vi "get_zero_crossings.vi"(9 "signal":dbl[](array[numeric]), 10 "index":dbl[](array[numeric])) -> (0 "size of p->n array":i32, 1 "size of n->p array":i32, 2 "p->n indexes":i32[](array[numeric]), 3 "n->p indexes":i32[](array[numeric]))   [LabVIEW 2019]
uses:
  <vilib>/ptbypt/NI_PtbyPt.lvlib
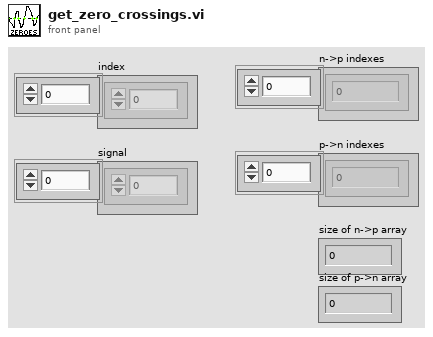
[diagram p1: front panel]
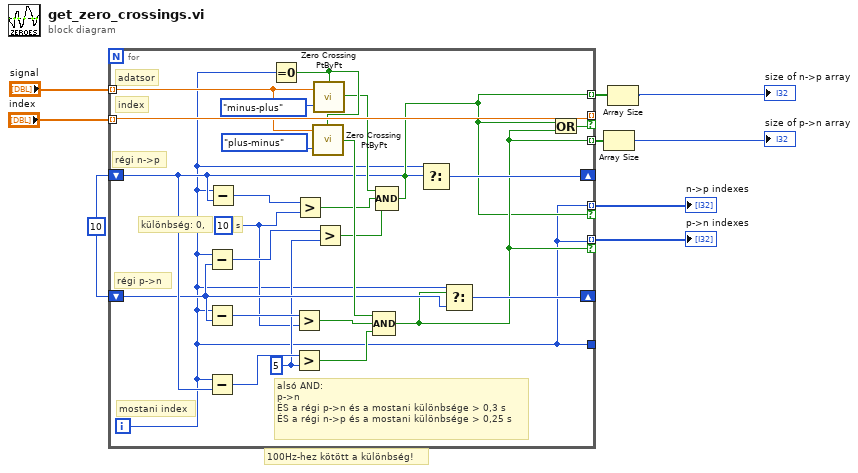
[diagram p0: block diagram]
diagram:
  w5 = 10
  # "100Hz-hez kötött a különbség!"
  n1 = for {
    tunnel: "signal" -> [w33] mode=indexing
    tunnel: "index" -> [w34] mode=indexing
    tunnel: [w34] -> _ mode=indexing if=w25
    tunnel: [w12] -> w2 mode=indexing
    tunnel: [w11] -> w6 mode=indexing
    shift-right: [w30] -> _
    shift-left: w5 -> [w21]
    shift-right: [w29] -> _
    shift-left: w5 -> [w17]
    tunnel: [w10] -> w7 mode=indexing if=w11
    tunnel: [w10] -> w8 mode=indexing if=w12
    tunnel: [w10] -> _
    i -> [w10]
    w14 = 5 ("y")
    w13 = 10
    # "adatsor"
    # "régi p->n"
    # "régi n->p"
    # "index"
    # "alsó AND:\np->n\nÉS a régi p->n és a mostani különbsége > 0,3 s\nÉS a régi n->p és a mostani különbsége > 0,25 s"
    # "mostani index"
    # "s"
    # "különbség: 0,"
    n2 = Subtract(x=w10, y=w17) -> (x-y=w18:i32)
    n3 = Subtract(x=w10, y=w17) -> (x-y=w22:i32)
    n4 = Subtract(x=w10, y=w21) -> (x-y=w15:i32)
    n5 = Subtract(x=w10, y=w21) -> (x-y=w24:i32)
    n6 = Equal To 0?(x=w10) -> (x = 0?=w28:bool)
    n7 = Greater?(x=w22, y=w13) -> (0:w20:bool)
    n8 = Greater?(x=w15, y=w14) -> (0:w19:bool)
    n9 = Greater?(x=w24, y=w13) -> (0:w23:bool)
    n10 = call <vilib>:"Zero Crossing PtByPt.vi"("initialize"=w28, "direction"=enum16{"either", "minus-plus", "plus-minus"}."plus-minus", "input data point"=w33) -> ("crossing"=w26:bool)
    n11 = call <vilib>:"Zero Crossing PtByPt.vi"("initialize"=w28, "direction"=enum16{"either", "minus-plus", "plus-minus"}."minus-plus", "input data point"=w33) -> ("crossing"=w27:bool)
    n12 = Greater?(x=w18, y=w14) -> (0:w16:bool)
    n13 = Compound Arithmetic op=AND(w26, w20, w19) -> (w12:bool)
    n14 = Compound Arithmetic op=AND(w27, w23, w16) -> (w11:bool)
    n15 = Select(t=w10, s=w11, f=w21) -> (s? t:f=w30:i32)
    n16 = Select(t=w10, s=w12, f=w17) -> (s? t:f=w29:i32)
    n17 = Or(x=w11, y=w12) -> (x .or. y?=w25:bool)
  }
  "p->n indexes" <- w8
  "n->p indexes" <- w7
  n18 = Array Size(array=w2) -> (size(s)=→"size of p->n array":i32)
  n19 = Array Size(array=w6) -> (size(s)=→"size of n->p array":i32)
